vi "CoreState_Stopped.vi"(8 "error in (no error)":errorcluster, 11 "launcher in":refnum<class "launcher.lvclass">) -> (0 "error out":errorcluster, 3 "launcher out":refnum<class "launcher.lvclass">)   [LabVIEW 2021, in "launcher.lvclass"]
uses:
  launcher.lvclass
  launcher.lvclass/launcher.ctl
  <vilib>/nisyscfg/Close (Hardware).vi
  <vilib>/nisyscfg/Close (System).vi
  <userlib>/S2 Labs/Module Framework/Modules/Base/Module.lvclass
  <userlib>/S2 Labs/Alarms and Events Toolkit/Alarms/Alarms Events.lvclass
  <vilib>/nisyscfg/nisyscfg.lvlib
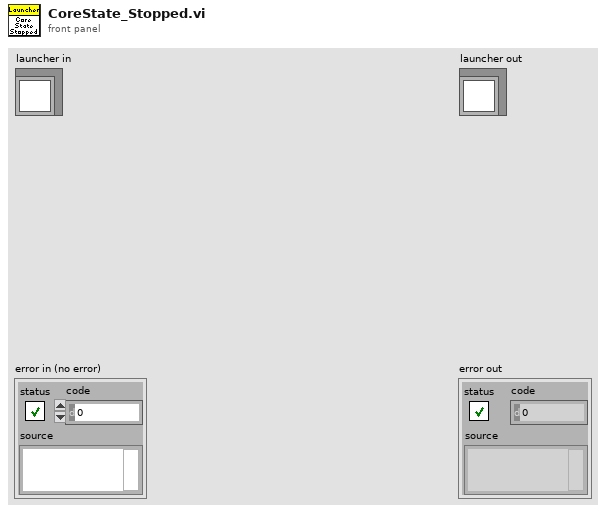
[diagram p1: front panel]
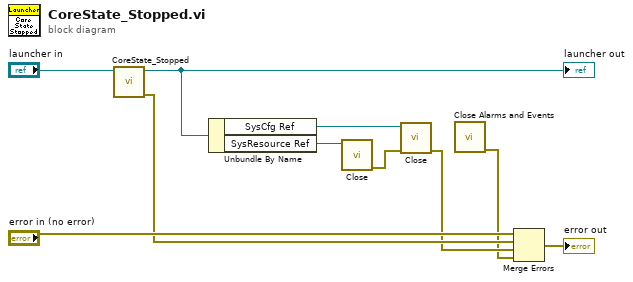
[diagram p0: block diagram]
diagram:
  n1 = call-parent "CoreState_Stopped.vi"("Module in"="launcher in") -> ("error out"=w3:errorcluster, "Module out"=w5:refnum<class "launcher.lvclass">)  [unwired: 9 in]
  "launcher out" <- w5
  n2 = Unbundle By Name(w5) -> ("SysCfg Ref"=w7:refnum<k21>, "SysResource Ref"=w6:refnum<k20>)
  n3 = call-poly <vilib>:"Close.vi"("Resource in"=w6) -> ("error out"=w8:errorcluster)  [unwired: 10 in]
  n4 = call-poly <vilib>:"Close.vi"("error in (no error)"=w8, "Session in"=w7) -> ("error out"=w2:errorcluster)  [unwired: 9 in]
  n5 = call <userlib>:"Close Alarms and Events.vi"() -> ("error out"=w1:errorcluster)  [unwired: 11 in]
  n6 = Merge Errors("error in (no error)", w3, w2, w1) -> (→"error out":errorcluster)
